vi "set_params.vi"(8 "error in (no error)":errorcluster caption="entrée d'erreur (pas d'erreur)", 11 "BayesianRidge.lvclass 2":refnum<class "BayesianRidge.lvclass">) -> (0 "error out":errorcluster caption="sortie d'erreur", 3 "BayesianRidge.lvclass":refnum<class "BayesianRidge.lvclass">)   [LabVIEW 2020, in "BayesianRidge.lvclass"]
uses:
  BayesianRidge.lvclass
  BayesianRidge.lvclass/BayesianRidge.ctl
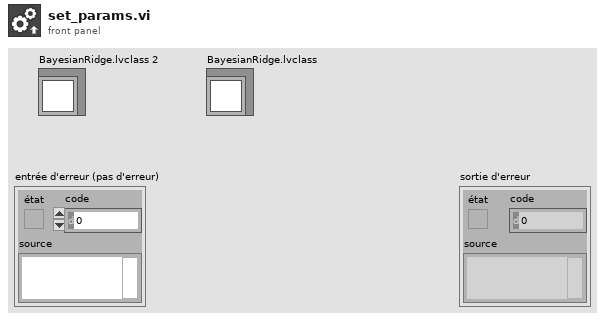
[diagram p1: front panel]
types:
  T1 = typedef "bayesian_ridge_params.ctl" = cluster{"n_iter":dbl, "tol":dbl, "alpha_1":dbl, "alpha_2":dbl, "lambda_1":dbl, "lambda_2":dbl, "alpha_init":cluster{"alpha_init_type":string, "alpha_init_float":dbl}, "lambda_init":cluster{"lambda_init_type":string, "lambda_init_float":dbl}, "compute_score":bool, "fit_intercept":bool, "normalize":bool, "copy_X":bool, "verbose":bool}
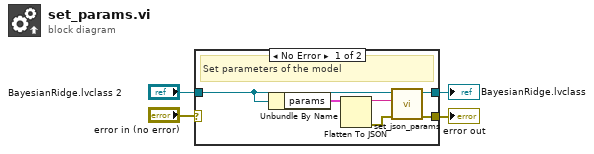
[diagram p0: block diagram]
diagram:
  n1 = case shown="No Error" "error in (no error)" {
    selector: "error in (no error)" -> [_ w12]
    tunnel: [w7 w12] -> w3
    tunnel: [w8 w11] -> w1
    tunnel: "BayesianRidge.lvclass 2" -> [w5 w11]
    frame No Error {
      # "Set parameters of the model"
      n2 = Unbundle By Name(w5) -> ("params"=w10:T1)
      n3 = Flatten To JSON(anything=w10) -> (JSON string=w9:string, 11:w6:errorcluster)  [unwired: 2 in]
      n4 = call-dynamic "set_json_params.vi"("error in (no error)"=w6, "params"=w9, "Model en entrée"=w5) -> ("error out"=w7:errorcluster, "Model en sortie"=w8:refnum<class "BayesianRidge.lvclass">)  [unwired: 7 in]
    }
    frame Error {
    }
  }
  "error out" <- w3
  "BayesianRidge.lvclass" <- w1
